vi "to_json.vi"(8 "error in":errorcluster, 11 "parquet in":refnum<class "parquet.lvclass">) -> (0 "error out":errorcluster, 2 "json":string, 3 "parquet out":refnum<class "parquet.lvclass">)   [LabVIEW 2020, in "datasources.lvlib" / "parquet.lvclass"]
uses:
  parquet.lvclass
  C:/code/labview-client/lv_src/Nominal Client/datasources/datasource/datasource.lvclass
  parquet.lvclass/parquet.ctl
  datasource/datasource.lvclass/datasource.ctl
  05961def-dca4-44fc-b9e8-664ec6be0171.vi
  932cd2f7-527d-47bd-aea7-c90cf7f59e63.vi
  datasource/source.get.vi
  datasource/target.get.vi
  <vilib>/JDP Science/JSONtext/Variant to JSON Text.vi
  <vilib>/JDP Science/JSONtext/support/Format JSON Object.vi
  timestampMetadata/timestampMetadata.lvclass
  nominal types/labels/labels.lvclass
  nominal types/properties/properties.lvclass
  <vilib>/JDP Science/JSONtext/LVClass Serializer/JSONtext LVClass Serializer.lvclass
  source/source.lvclass
  target/target.lvclass
  <vilib>/JDP Science/JSONtext/JSONtext.lvlib
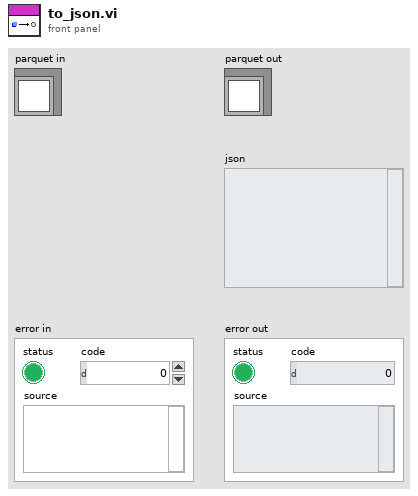
[diagram p1: front panel]
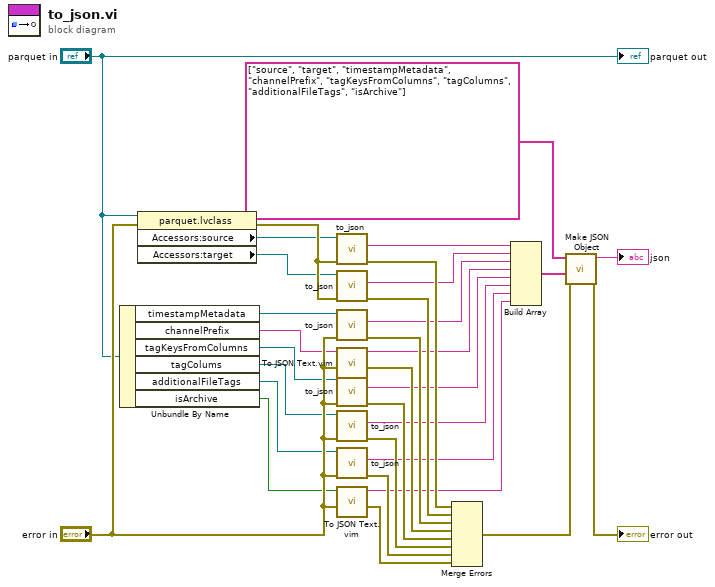
[diagram p0: block diagram]
diagram:
  n1 = Unbundle By Name("parquet in") -> ("timestampMetadata"=w17:refnum<class "timestampMetadata.lvclass">, "channelPrefix"=w22:string, "tagKeysFromColumns"=w19:refnum<class "labels.lvclass">, "tagColums"=w18:refnum<class "properties.lvclass">, "additionalFileTags"=w20:refnum<class "properties.lvclass">, "isArchive"=w21:bool)
  n2 = property class="parquet.lvclass"(reference="parquet in", error in="error in") -> (error out=w32:errorcluster, "Accessors:source"=w15:refnum<class "source.lvclass">, "Accessors:target"=w14:refnum<class "target.lvclass">)  [unwired: 1 out]
  n3 = call-dynamic "to_json.vi"("error in"=w32, "source in"=w15) -> ("error out"=w30:errorcluster, "json"=w13:string)  [unwired: 7 in, 1 out]
  n4 = call-dynamic "to_json.vi"("error in"=w32, "target in"=w14) -> ("error out"=w29:errorcluster, "json"=w12:string)  [unwired: 7 in, 1 out]
  n5 = call-dynamic "to_json.vi"("error in"="error in", "timestampMetadata in"=w17) -> ("error out"=w28:errorcluster, "json"=w11:string)  [unwired: 7 in, 1 out]
  n6 = call "To JSON Text.vim"("error in (no error)"="error in", "Anything"=w22) -> ("error out"=w27:errorcluster, "<JSON>"=w10:string)  [unwired: 8 in]
  n7 = call-dynamic "to_json.vi"("error in"="error in", "labels in"=w19) -> ("error out"=w26:errorcluster, "json"=w9:string)  [unwired: 7 in, 1 out]
  n8 = call-dynamic "to_json.vi"("error in"="error in", "properties in"=w18) -> ("error out"=w25:errorcluster, "json"=w8:string)  [unwired: 7 in, 1 out]
  n9 = call-dynamic "to_json.vi"("error in"="error in", "properties in"=w20) -> ("error out"=w24:errorcluster, "json"=w7:string)  [unwired: 7 in, 1 out]
  n10 = call "To JSON Text.vim"("error in (no error)"="error in", "Anything"=w21) -> ("error out"=w23:errorcluster, "<JSON>"=w6:string)  [unwired: 8 in]
  n11 = Merge Errors(w30, w29, w28, w27, w26, w25, w24, w23) -> (w2:errorcluster)
  n12 = Build Array(w13, w12, w11, w10, w9, w8, w7, w6) -> (w5:string[])
  n13 = call <vilib>:"Make JSON Object.vi"("error in (no error)"=w2, "JSON Items"=w5, "Item Names"=string[] ["source", "target", "timestampMetadata", "channelPrefix", "tagKeysFromColumns", "tagColumns", "additionalFileTags", "isArchive"]) -> ("error out"=→"error out":errorcluster, "<JSON>"=→"json":string)  [unwired: 7 in]
  "parquet out" <- "parquet in"
